vi "DFD FXP MRate Simulation.vi"   [LabVIEW 2017, in "NI_DigFilterLicensed.lvlib"]
doc: "Simulates the filtering process of a fixed-point multirate filter continuously. Wire data to the <B>signal in</B> input to determine the polymorphic instance to use or manually select the instance."
uses:
  <vilib>/addons/Digital Filter Design/NI_DigFilterLicensed.lvlib
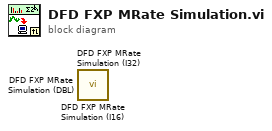
[diagram p0: block diagram]
diagram:
  n1 = call <vilib>:"DFD FXP MRate Simulation (I16).vi"() -> ()  [unwired: 9 in, 3 out]
  n2 = call <vilib>:"DFD FXP MRate Simulation (I32).vi"() -> ()  [unwired: 9 in, 3 out]
  n3 = call <vilib>:"DFD FXP MRate Simulation (DBL).vi"() -> ()  [unwired: 9 in, 3 out]
